vi "fwd-navx (SubVI).vi"(8 "error in (no error)":errorcluster, 9 "I2C Ref Out":T1, 10 "R_PWM":refnum<vi>, 11 "L_PWM":refnum<vi>) -> (0 "error out":errorcluster, 2 "I2C Ref Out out":T1, 3 "value Z":ext, 4 "Right+":bool, 6 "Left+":bool)   [LabVIEW 2017]
uses:
  <vilib>/myRIO/Instrument Drivers/Onboard IO/I2C/typedefs/I2C Reference.ctl
  <vilib>/myRIO/Common/Instrument Driver Framework/Utilities/typedefs/myRIO Generic Hardware Reference.ctl
  <vilib>/myRIO/Common/Instrument Driver Framework/Utilities/typedefs/Hardware Version Enum.ctl
  <vilib>/myRIO/Common/Instrument Driver Framework/Utilities/typedefs/myRIO v1.0 Reference.ctl
  <vilib>/myRIO/Common/Instrument Driver Framework/Utilities/typedefs/Generic FPGA Reference.ctl
  <vilib>/myRIO/Common/Instrument Driver Framework/myRIO v1.0/I2C/typedefs/I2C Channels Enum.ctl
  <vilib>/myRIO/Instrument Drivers/Onboard IO/I2C/typedefs/I2C Configuration.ctl
  <vilib>/myRIO/Instrument Drivers/Onboard IO/I2C/typedefs/I2C Transfer Rate.ctl
  <vilib>/myRIO/Instrument Drivers/Onboard IO/I2C/I2C.lvlib
panel:
  out "L":dbl
  out "R":dbl
  in  "accuracy":ext=5.0 format="%#_13g"
  in  "def PWM":ext=50.0 format="%#_13g"
  out "def Z":ext
  out "x-y":ext
  in  "offset":ext
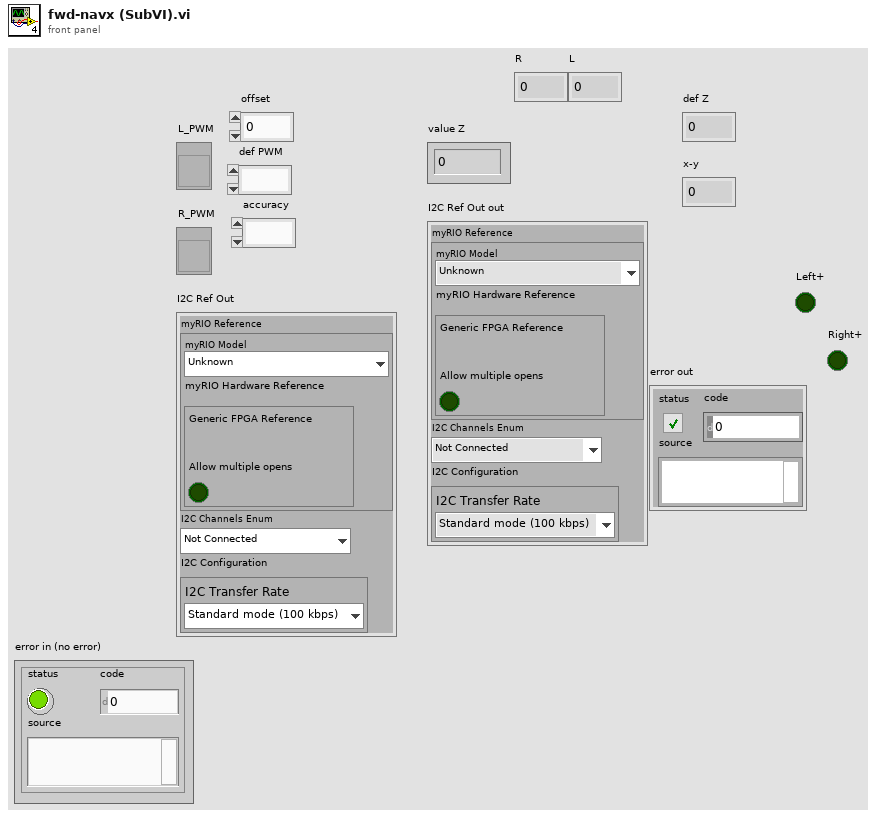
[diagram p1: front panel]
types:
  T1 = typedef "I2C.lvlib/I2C Reference.ctl" = cluster{"myRIO Reference":T2, "I2C Channels Enum":T6, "I2C Configuration":T7}
  T2 = typedef "myRIO Generic Hardware Reference.ctl" = cluster{"myRIO Model":T3, "myRIO Hardware Reference":T4}
  T3 = typedef "Hardware Version Enum.ctl" = enum16{"Unknown", "myRIO-1900", "myRIO-1950", "roboRIO", "NI ELVIS RIO CM"}
  T4 = typedef "myRIO v1.0 Reference.ctl" = cluster{"Generic FPGA Reference":T5, "Allow multiple opens":bool}
  T5 = typedef "Generic FPGA Reference.ctl" = refnum<k20>
  T6 = typedef "I2C Channels Enum.ctl" = enum16{"Not Connected", "A/I2C", "B/I2C", "I2C/I2C"}
  T7 = typedef "I2C.lvlib/I2C Configuration.ctl" = cluster{"I2C Transfer Rate":T8}
  T8 = typedef "I2C.lvlib/I2C Transfer Rate.ctl" = enum16{"Standard mode (100 kbps)", "Fast mode (400 kbps)"}
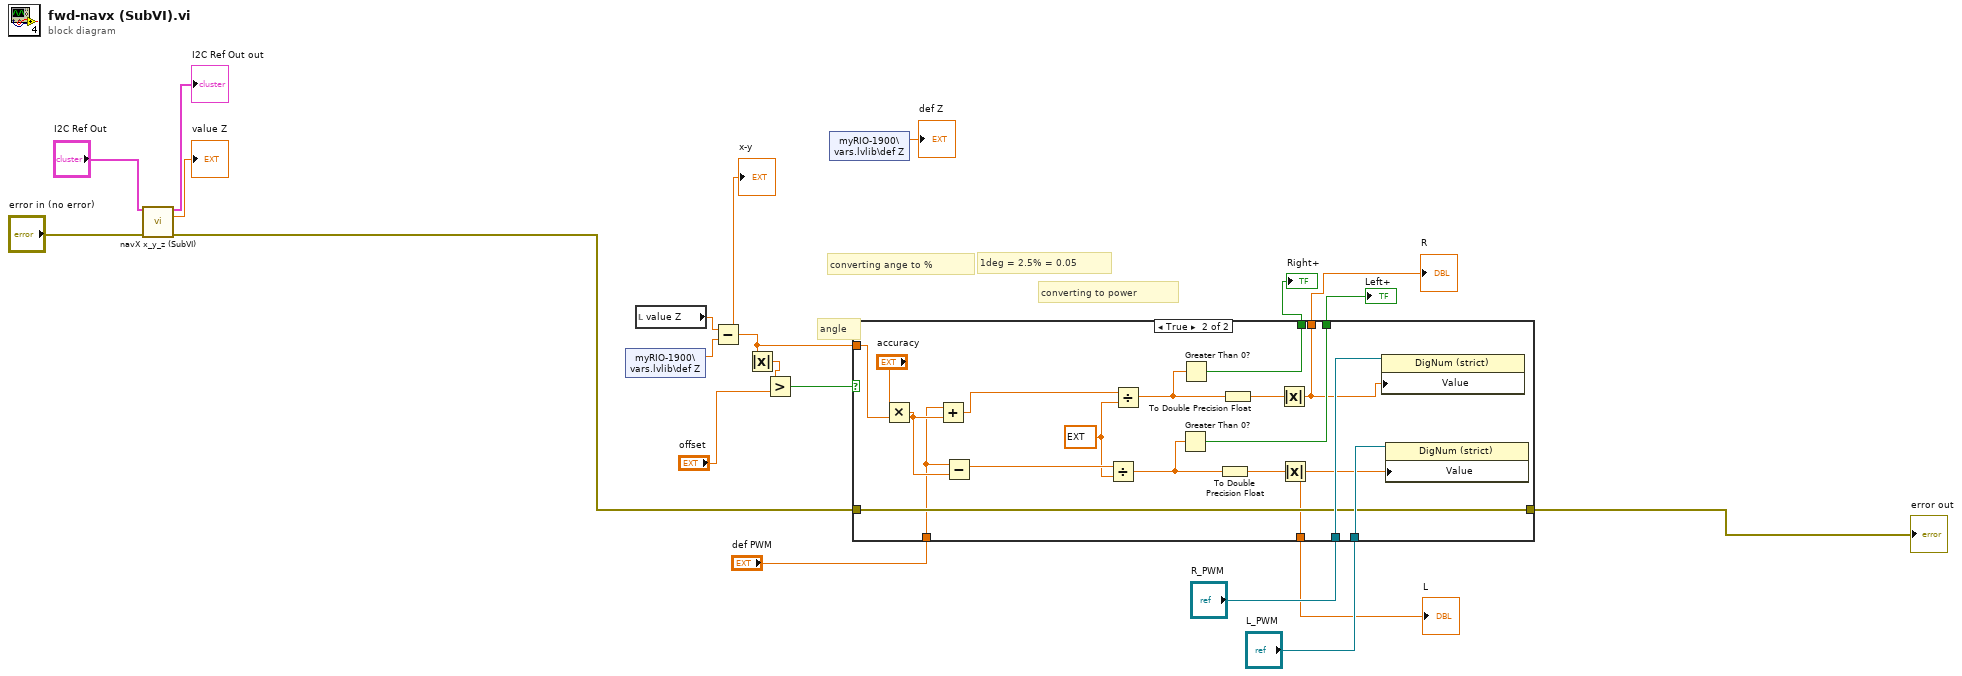
[diagram p0: block diagram]
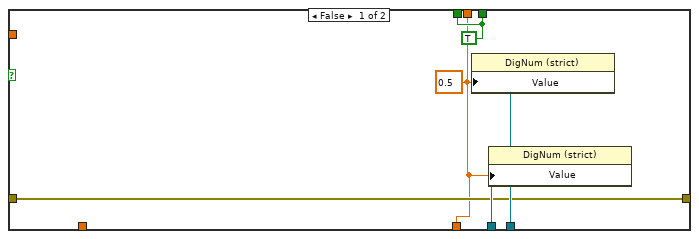
[diagram p2: hidden frame]
diagram:
  # "converting to power"
  # "converting ange to %"
  # "angle"
  # "1deg = 2.5% = 0.05"
  n1 = call "navX x_y_z (SubVI).vi"("I2C Ref Out in"="I2C Ref Out", "error in (no error)"="error in (no error)") -> ("I2C Ref Out out"=→"I2C Ref Out out":T1, "value Z"=→"value Z":ext, "error out"=w3:errorcluster)  [unwired: 9 in, 2 out]
  n2 = shared-variable "myRIO-1900\\vars.lvlib\\def Z"() -> (w1:ext)  [unwired: 1 in, 1 out]
  n3 = local read "value Z"() -> (w18:ext)
  n4 = Subtract(x=w18, y=w1) -> (x-y=w13:ext)
  "x-y" <- w13
  n5 = Absolute Value(x=w13) -> (abs(x)=w15:ext)
  n6 = Greater?(x=w15, y="offset") -> (0:w17:bool)
  n7 = shared-variable "myRIO-1900\\vars.lvlib\\def Z"() -> (→"def Z":ext)  [unwired: 1 in, 1 out]
  n8 = case shown="True" w17 {
    tunnel: "R_PWM" -> [w24 w42]
    tunnel: "L_PWM" -> [w25 w43]
    tunnel: [w23 w41] -> w6
    tunnel: w3 -> [w23 w41]
    tunnel: w13 -> [_ w40]
    tunnel: "def PWM" -> [_ w32]
    tunnel: [w22 w29] -> w11
    tunnel: [w22 w28] -> w10
    tunnel: [w21 w27] -> w5
    tunnel: [w21 w26] -> w4
    frame False {
      w22 = TRUE
      w21 = 0.5 ("Value")
      n9 = property class="DigNum (strict)"(reference=w25, "Value"=w21) -> ()  [unwired: 1 in, 2 out]
      n10 = property class="DigNum (strict)"(reference=w24, "Value"=w21) -> ()  [unwired: 1 in, 2 out]
    }
    frame True {
      w35 = ext 100.0 ("y")
      n11 = Multiply(x="accuracy", y=w40) -> (x*y=w38:ext)
      n12 = Add(x=w32, y=w38) -> (x+y=w36:ext)
      n13 = Subtract(x=w32, y=w38) -> (x-y=w37:ext)
      n14 = Divide(x=w37, y=w35) -> (x/y=w30:ext)
      n15 = Divide(x=w36, y=w35) -> (x/y=w31:ext)
      n16 = Greater Than 0?(x=w30) -> (x > 0?=w28:bool)
      n17 = Greater Than 0?(x=w31) -> (x > 0?=w29:bool)
      n18 = To Double Precision Float(number=w30) -> (double precision float=w33:dbl)
      n19 = To Double Precision Float(number=w31) -> (double precision float=w34:dbl)
      n20 = Absolute Value(x=w34) -> (abs(x)=w27:dbl)
      n21 = Absolute Value(x=w33) -> (abs(x)=w26:dbl)
      n22 = property class="DigNum (strict)"(reference=w42, "Value"=w27) -> ()  [unwired: 1 in, 2 out]
      n23 = property class="DigNum (strict)"(reference=w43, "Value"=w26) -> ()  [unwired: 1 in, 2 out]
    }
  }
  "Right+" <- w11
  "Left+" <- w10
  "error out" <- w6
  "R" <- w5
  "L" <- w4
